vi "Graph Cursor Update.vi"(7 "Action":enum16{"Reset", "Update"}(ring)=enum."Update", 8 "error in":errorcluster, 9 "New X position":dbl, 10 "Cursor Type":enum16{"Movable", "Fixed", "All"}(ring), 11 "Graph Refs in":refnum<vi>[](array[refnum])) -> (0 "error out":errorcluster, 3 "Graph Refs out":refnum<vi>[](array[refnum]))   [LabVIEW 2023, in "FPT Intermodulation UI.lvlib"]
doc: "Use this VI to update the cursor positions on the selected graphs according to the selected cursor type.\n\nFor fixed cursor creation, ensure that its name contains the word ‘fix’. \n\nAll default cursors are treated as movable cursors."
uses:
  FPT Intermodulation UI.lvlib
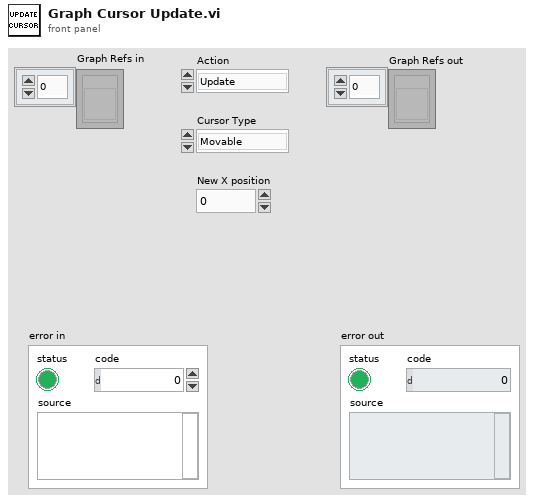
[diagram p1: front panel]
types:
  T1 = typedef "LVCursorListTypeDef.ctl" = cluster{"Name":string, "Color":u32, "Style":u8, "Point Style":u8, "Name Visible":bool, "Allow Drag":bool, "Cursor Mode":u32, "Plot":i32, "Index":i32, "Position":cluster{"X":dbl, "Y":dbl}, "X Scale":u32, "Y Scale":u32, "Watch Plots":i32[], "Watch All Plots":bool, "Plot Area":i32, "Label Offset":cluster{"X":dbl, "Y":dbl}}[]
  T2 = cluster{"Name":string, "Color":u32, "Style":u8, "Point Style":u8, "Name Visible":bool, "Allow Drag":bool, "Cursor Mode":u32, "Plot":i32, "Index":i32, "Position":cluster{"X":dbl, "Y":dbl}, "X Scale":u32, "Y Scale":u32, "Watch Plots":i32[], "Watch All Plots":bool, "Plot Area":i32, "Label Offset":cluster{"X":dbl, "Y":dbl}}
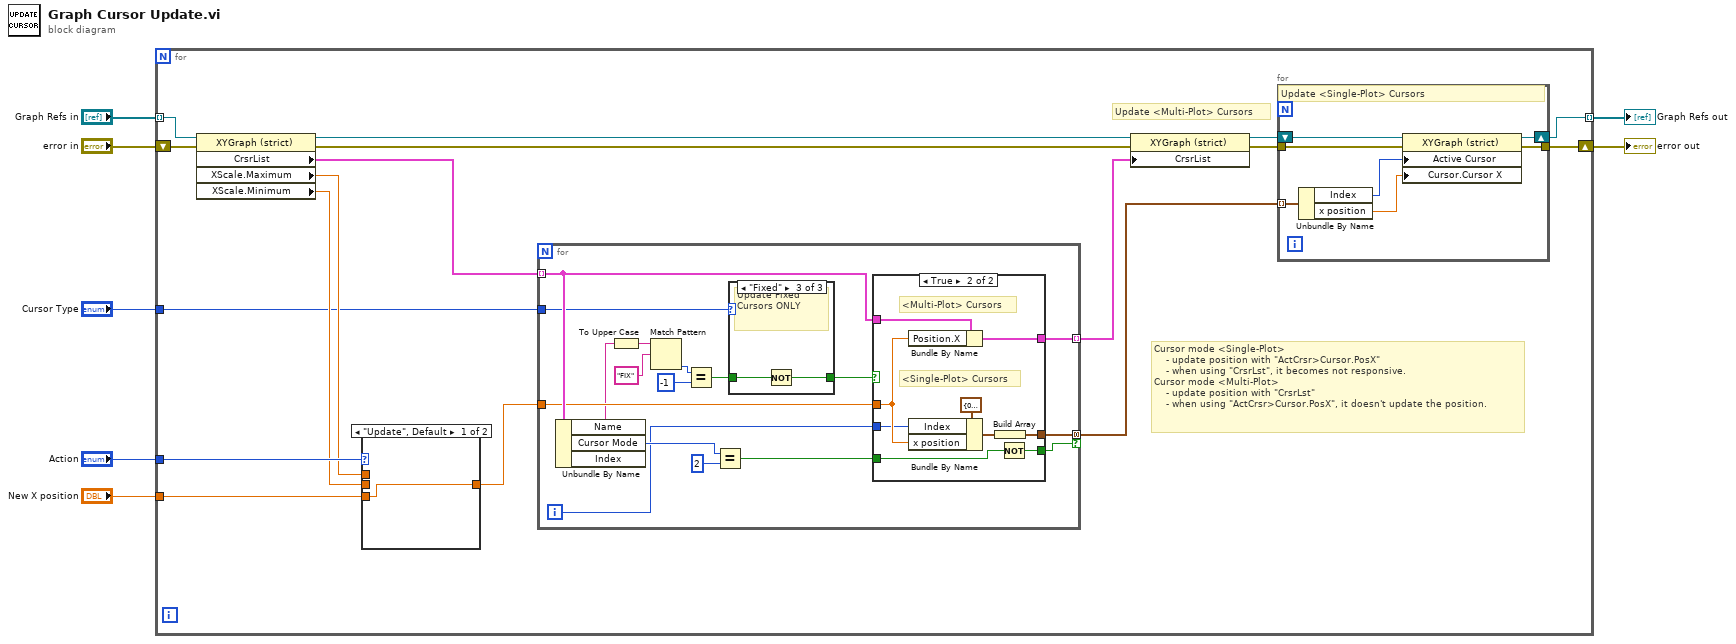
[diagram p0: block diagram]
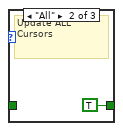
[diagram p3: hidden frame]
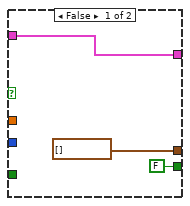
[diagram p4: hidden frame]
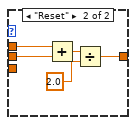
[diagram p5: hidden frame]
diagram:
  n1 = for {
    tunnel: "Graph Refs in" -> [w10] mode=indexing
    shift-right: [w12] -> w1
    shift-left: "error in" -> [w22]
    tunnel: [w8] -> w6 mode=indexing
    tunnel: "Action" -> [w20]
    tunnel: "New X position" -> [w17]
    tunnel: "Cursor Type" -> [w11]
    # "Update <Multi-Plot> Cursors"
    # "Cursor mode <Single-Plot>\n    - update position with \"ActCrsr>Cursor.PosX\"\n    - when using \"CrsrLst\", it becomes not responsive.\nCursor mode <Multi-Plot>\n    - update position with \"CrsrLst\"\n    - when using \"ActCrsr>Cursor.PosX\", it doesn't update the position."
    n2 = property on="Property Node" class="XYGraph (strict)"(reference=w10, error in=w22) -> (reference out=w23:refnum<vi>, error out=w24:errorcluster, "CrsrList"=w21:T1, "XScale.Maximum"=w19:dbl, "XScale.Minimum"=w18:dbl)
    n3 = case shown="\"Update\", Default" w20 {
      tunnel: w19 -> [_ w70]
      tunnel: w18 -> [_ w69]
      tunnel: w17 -> [w65 _]
      tunnel: [w65 w66] -> w16
      frame "Update", Default {
      }
      frame "Reset" {
        n4 = Add(x=w70, y=w69) -> (x+y=w67:dbl)
        n5 = Divide(x=w67, y=2.0) -> (x/y=w66:dbl)
      }
    }
    n6 = for {
      tunnel: w21 -> [w47] mode=indexing
      tunnel: w16 -> [w45]
      tunnel: [w48] -> w15 mode=indexing
      tunnel: [w46] -> w9 mode=concatenating if=w34
      tunnel: w11 -> [w38]
      i -> [w36]
      n7 = Unbundle By Name(w47) -> ("Name"=w33:string, "Cursor Mode"=w44:u32)  [unwired: 1 out]
      n8 = To Upper Case(1:w33) -> (0:w41:string)
      n9 = Match Pattern(string=w41, regular expression="FIX") -> (offset past match=w40:i32)  [unwired: 1 in, 3 out]
      n10 = Equal?(x=w40, y=-1) -> (x = y?=w37:bool)
      n11 = Equal?(x=w44, y=u32 2) -> (x = y?=w35:bool)
      n12 = case shown="\"Fixed\"" w38 {
        tunnel: w37 -> [w49 _ w52]
        tunnel: [w49 TRUE w51] -> w32
        frame "Movable", Default {
          # "Update Movable Cursors ONLY"
        }
        frame "All" {
          # "Update ALL Cursors"
        }
        frame "Fixed" {
          # "Update Fixed Cursors ONLY"
          n13 = Not(x=w52) -> (.not. x?=w51:bool)
        }
      }
      n14 = case shown="True" w32 {
        tunnel: [w54 w61] -> w48
        tunnel: w47 -> [w54 w57]
        tunnel: [cluster{"Index":i32, "x position":dbl}[] [] w62] -> w46
        tunnel: w45 -> [_ w64]
        tunnel: w36 -> [_ w63]
        tunnel: w35 -> [_ w58]
        tunnel: [FALSE w56] -> w34
        frame False {
        }
        frame True {
          # "<Single-Plot> Cursors"
          # "<Multi-Plot> Cursors"
          n15 = Bundle By Name(cluster=w57, "Position.X"=w64) -> (w61:T2)
          n16 = Bundle By Name(cluster=cluster{"Index":i32, "x position":dbl} {"Index"=0, "x position"=0.0}, "Index"=w63, "x position"=w64) -> (w59:cluster{"Index":i32, "x position":dbl})
          n17 = Build Array(w59) -> (w62:cluster{"Index":i32, "x position":dbl}[])
          n18 = Not(x=w58) -> (.not. x?=w56:bool)
        }
      }
    }
    n19 = property on="Property Node" class="XYGraph (strict)"(reference=w23, error in=w24, "CrsrList"=w15) -> (reference out=w14:refnum<vi>, error out=w13:errorcluster)
    n20 = for {
      tunnel: w9 -> [w27] mode=indexing
      tunnel: w13 -> [w30]
      tunnel: [w28] -> w12
      shift-right: [w29] -> w8
      shift-left: w14 -> [w31]
      # "Update <Single-Plot> Cursors"
      n21 = Unbundle By Name(w27) -> ("Index"=w26:i32, "x position"=w25:dbl)
      n22 = property on="Property Node" class="XYGraph (strict)"(reference=w31, error in=w30, "Active Cursor"=w26, "Cursor.Cursor X"=w25) -> (reference out=w29:refnum<vi>, error out=w28:errorcluster)
    }
  }
  "Graph Refs out" <- w6
  "error out" <- w1
